vi "getSomeVideo.vi"(8 "error in (no error)":errorcluster, 11 "videoId":string) -> (0 "error out":errorcluster, 3 "Video out":refnum<class "Video.lvclass">)   [LabVIEW 2017, in "ThirdPartyYoutubeClass.lvclass"]
uses:
  ThirdPartyYoutubeClass.lvclass
  Video Class/Video.lvclass
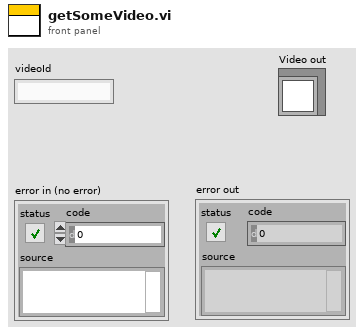
[diagram p1: front panel]
types:
  T1 = enum16{"Create", "Get Reference", "Print", "Close"}
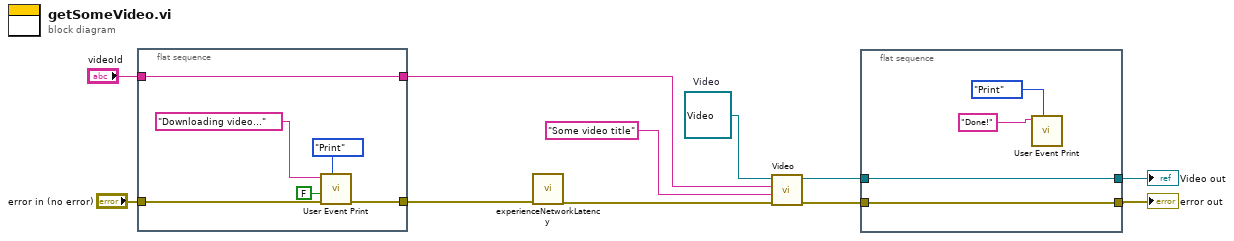
[diagram p0: block diagram]
diagram:
  w1 = refnum<class "Video.lvclass"> refnum  # Video
  n1 = flat-sequence {
    tunnel: "error in (no error)" -> [w17]
    tunnel: [w15] -> w10
    tunnel: "videoId" -> [w16]
    tunnel: [w16] -> w8
    frame #0 {
      n2 = call "User Event Print.vi"("Options"=T1."Print", "error in (no error)"=w17, "add EOL? (T)"=FALSE, "String to Print"="Downloading video..." ("ConsoleOut")) -> ("error out"=w15:errorcluster)  [unwired: 6 in, 1 out]
    }
  }
  n3 = call "experienceNetworkLatency.vi"("error in (no error)"=w10) -> ("error out"=w6:errorcluster)  [unwired: 10 in]
  n4 = call "Video.vi"("error in (no error)"=w6, "title"="Some video title", "id"=w8, "Video in"=w1) -> ("error out"=w5:errorcluster, "Video out"=w3:refnum<class "Video.lvclass">)  [unwired: 6 in]
  n5 = flat-sequence {
    tunnel: w5 -> [w21]
    tunnel: [w21] -> w4
    tunnel: w3 -> [w20]
    tunnel: [w20] -> w2
    frame #0 {
      n6 = call "User Event Print.vi"("Options"=T1."Print", "String to Print"="Done!" ("ConsoleOut")) -> ()  [unwired: 8 in, 2 out]
    }
  }
  "error out" <- w4
  "Video out" <- w2
